vi "Clean images.vi"(11 "html in":string="sdfsfsse") -> (0 "after hyperlink":string, 1 "image data":T1, 2 "link":string, 3 "before hyperlink":string, 4 "Success?":bool)   [LabVIEW 2019]
uses:
  <vilib>/picture/picture.llb/imagedata.ctl
panel:
  out "output cluster":T2
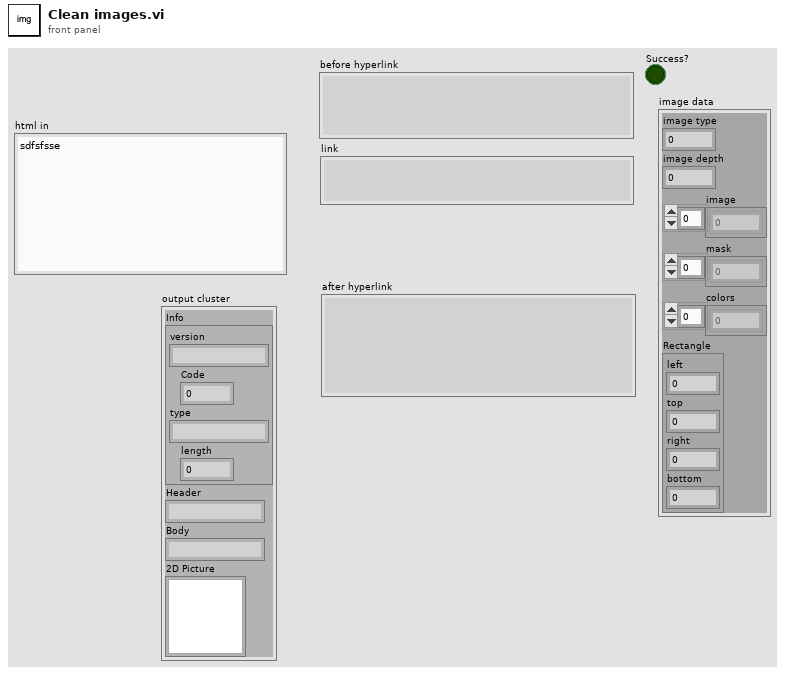
[diagram p1: front panel]
types:
  T1 = typedef "imagedata.ctl" = cluster{"image type":i32, "image depth":i32, "image":u8[], "mask":u8[], "colors":u32[], "Rectangle":cluster{"left":i16, "top":i16, "right":i16, "bottom":i16}}
  T2 = cluster{"Info":cluster{"version":string, "Code":i32, "type":string, "length":i32}, "Header":string, "Body":string, "2D Picture":picture}
  T3 = cluster{"Info":cluster{"version":string, "Code":i32, "type":string, "length":i32}, "Header":string, "Body":string}
  T4 = cluster{"version":string, "Code":i32, "type":string, "length":i32}
  T5 = cluster{"Info":cluster{"version":string, "Code":i32, "type":string, "length":i32}, "Header":string, "Body":string, "new picture":picture}
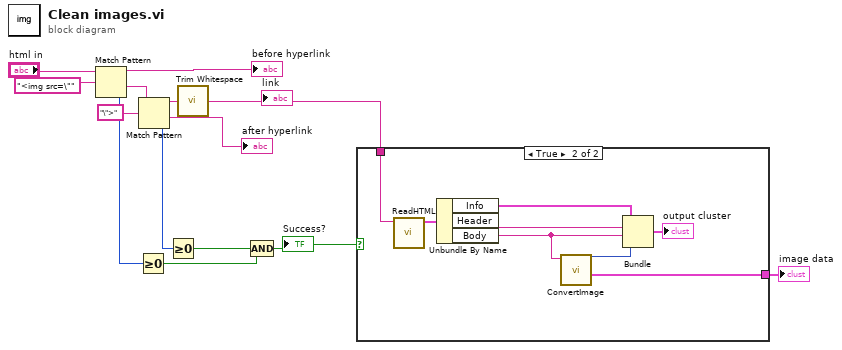
[diagram p0: block diagram]
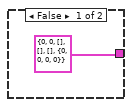
[diagram p2: hidden frame]
diagram:
  n1 = Match Pattern(string="html in", regular expression="<img src=\"" ("format string")) -> (before substring=→"before hyperlink":string, after substring=w12:string, offset past match=w8:i32)  [unwired: 1 in, 1 out]
  n2 = Greater Or Equal To 0?(x=w8) -> (x >= 0?=w5:bool)
  n3 = Match Pattern(string=w12, regular expression="\">" ("format string")) -> (before substring=w10:string, after substring=→"after hyperlink":string, offset past match=w7:i32)  [unwired: 1 in, 1 out]
  n4 = Greater Or Equal To 0?(x=w7) -> (x >= 0?=w6:bool)
  n5 = call <vilib>:"Trim Whitespace.vi"("string"=w10) -> ("trimmed string"=w3:string)  [unwired: 1 in]
  "link" <- w3
  n6 = Compound Arithmetic op=AND(w6, w5) -> (w2:bool)
  "Success?" <- w2
  n7 = case shown="True" w2 {
    tunnel: w3 -> [_ w19]
    tunnel: [T1 {"image type"=0, "image depth"=0, "image"=[], "mask"=[], "colors"=[], "Rectangle"={"left"=0, "top"=0, "right"=0, "bottom"=0}} ("image data") w16] -> w1
    frame False {
    }
    frame True {
      n8 = call "ReadHTML.vi"("url"=w19) -> ("Info"=w20:T3)  [unwired: 8 in, 2 out]
      n9 = Unbundle By Name(w20) -> ("Info"=w21:T4, "Header"=w23:string, "Body"=w22:string)
      n10 = call "ConvertImage.vi"("body"=w22) -> ("image data"=w16:T1, "new picture"=w17:picture)  [unwired: 9 in]
      n11 = Bundle("Info"=w21, "Header"=w23, "Body"=w22, "new picture"=w17) -> (→"output cluster":T5)  [unwired: 1 in]
    }
  }
  "image data" <- w1
